vi "PH_AWG-510.Init.vi"(0 "VI in":refnum<vi>, 5 "error in (no error)":errorcluster) -> (14 "VI out":refnum<vi>, 19 "error out":errorcluster)   [LabVIEW 2014, in "PH_AWG-510.lvlib"]
doc: "tis opens a VISA session, gets the settings of the hardware, stores these at own attributes and displays them at the GUI."
uses:
  PH_AWG-510.lvlib
  instr.lib/awg510/Tektronix AWG510 - Driver.lvlib
  PH_Common/PH_Common.lvlib
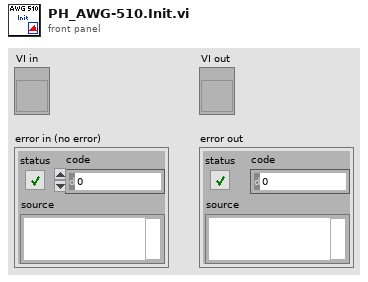
[diagram p1: front panel]
types:
  T1 = typedef "PH_AWG-510.lvlib/PH_AWG-510.i attribute.ctl" = cluster{"GUI Refs":cluster{"Delete":refnum<vi>, "Trigger Settings":refnum<vi>, "Start Device":refnum<vi>, "Instrument Information":refnum<vi>, "Lock Frontpanel":refnum<vi>, "Waveform Pattern File":refnum<vi>, "Initialize":refnum<vi>, "Output Settings":refnum<vi>}, "Instrument Information":T2, "Initialized?":bool, "Current Settings":cluster{"Trigger":T3, "Output Settings":T4}, "Wanted Settings":cluster{"Trigger":T3, "Output Settings":T4}, "Device frontpanel locked?":bool, "Default File Path":path}
  T2 = typedef "PH_AWG-510.lvlib/PH_AWG-510.Instrument Information Dataset.ctl" = cluster{"VISA resource name":refnum<visa-resource-name>, "Instrument Firmware Revision":string, "Manufacturer":string, "Model":string, "Serial Number":string, "Error Message":string, "Device Status":enum16{"stopped", "wating for trigger", "running", "Failure"}}
  T3 = typedef "PH_AWG-510.lvlib/PH_AWG-510.Trigger Settings.ctl" = cluster{"Mode":enum16{"Continuous", "Triggered", "Gated", "Enhanced"}, "Level (V)":dbl, "External Source":bool}
  T4 = typedef "PH_AWG-510.lvlib/PH_AWG-510.Output Settings.ctl" = cluster{"Activate Channel":bool, "VPP (V)":dbl, "Clock (Hz)":dbl, "File Name (Device)":string, "#1":u16, "#2":u16, "#3":u16, "#4":u16, "#5":u16, "#6":u16, "#7":u16, "#8":u16, "#9":u16, "#10":u16, "#11":u16, "#12":u16, "#13":u16, "#14":u16, "#15":u16, "#16":u16, "#17":u16, "#18":u16, "#19":u16, "#20":u16, "Offset (V)":dbl}
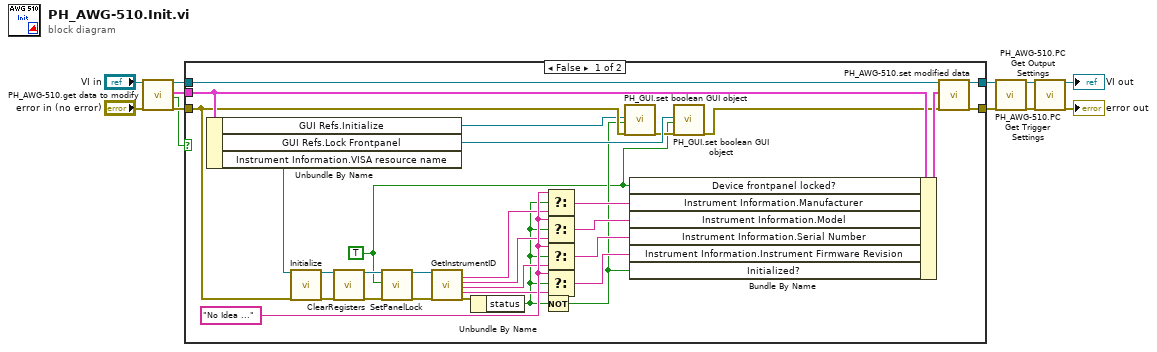
[diagram p0: block diagram]
diagram:
  n1 = call "PH_AWG-510.get data to modify.vi"("i ref in"="VI in", "error in (no error)"="error in (no error)") -> ("i ref out"=w10:refnum<vi>, "i attribute"=w8:T1, "timed out"=w7:bool, "error out"=w9:errorcluster)  [unwired: 14 in]
  n2 = case shown="False" w7 {
    tunnel: [w42 w43] -> w6
    tunnel: w10 -> [w41 w44]
    tunnel: [w40 w44] -> w4
    tunnel: w9 -> [w17 w43]
    tunnel: w8 -> [w38 _]
    frame False {
      w13 = TRUE ("Status (Lock)")
      w32 = "No Idea ..."
      n3 = Unbundle By Name(w38) -> ("GUI Refs.Initialize"=w15:refnum<vi>, "GUI Refs.Lock Frontpanel"=w30:refnum<vi>, "Instrument Information.VISA resource name"=w33:refnum<visa-resource-name>)
      n4 = call "Initialize.vi"("VISA resource name"=w33, "error in (no error)"=w17) -> ("VISA resource name out"=w29:refnum<visa-resource-name>, "error out"=w28:errorcluster)  [unwired: 16 in]
      n5 = call "ClearRegisters.vi"("VISA resource name"=w29, "error in (no error)"=w28) -> ("VISA resource name out"=w20:refnum<visa-resource-name>, "error out"=w22:errorcluster)  [unwired: 16 in]
      n6 = call "SetPanelLock.vi"("VISA resource name"=w20, "Status (Lock)"=w13, "error in"=w22) -> ("VISA resource name out"=w19:refnum<visa-resource-name>, "error out"=w21:errorcluster)  [unwired: 15 in]
      n7 = call "GetInstrumentID.vi"("VISA resource name"=w19, "error in"=w21) -> ("Manufacturer"=w26:string, "Model"=w25:string, "Serial Number"=w23:string, "Instrument Firmware Revision"=w24:string, "error out"=w27:errorcluster)  [unwired: 12 in, 1 out]
      n8 = Unbundle By Name(w27) -> ("status"=w18:bool)
      n9 = Not(x=w18) -> (.not. x?=w14:bool)
      n10 = Select(t=w32, s=w18, f=w26) -> (s? t:f=w37:string)
      n11 = Select(t=w32, s=w18, f=w25) -> (s? t:f=w36:string)
      n12 = Select(t=w32, s=w18, f=w23) -> (s? t:f=w34:string)
      n13 = Select(t=w32, s=w18, f=w24) -> (s? t:f=w35:string)
      n14 = call "PH_GUI.set boolean GUI object.vi"("Boolean Knob GUI Ref"=w15, "Value"=w14, "error in (no error)"=w17) -> ("error out"=w16:errorcluster)  [unwired: 16 in]
      n15 = Bundle By Name(cluster=w38, "Device frontpanel locked?"=w13, "Instrument Information.Manufacturer"=w37, "Instrument Information.Model"=w36, "Instrument Information.Serial Number"=w34, "Instrument Information.Instrument Firmware Revision"=w35, "Initialized?"=w14) -> (w39:T1)
      n16 = call "PH_GUI.set boolean GUI object.vi"("Boolean Knob GUI Ref"=w30, "Value"=w13, "error in (no error)"=w16) -> ("error out"=w31:errorcluster)  [unwired: 16 in]
      n17 = call "PH_AWG-510.set modified data.vi"("i ref in"=w41, "i attribute"=w39, "error in (no error)"=w31) -> ("i ref out"=w40:refnum<vi>, "error out"=w42:errorcluster)  [unwired: 15 in]
    }
    frame True {
    }
  }
  n18 = call "PH_AWG-510.PC Get Trigger Settings.vi"("VI in"=w4, "error in (no error)"=w6) -> ("VI out"=w3:refnum<vi>, "error out"=w5:errorcluster)  [unwired: 16 in]
  n19 = call "PH_AWG-510.PC Get Output Settings.vi"("VI in"=w3, "error in (no error)"=w5) -> ("VI out"=→"VI out":refnum<vi>, "error out"=→"error out":errorcluster)  [unwired: 16 in]
